vi "Image to base64_v2.vi"() -> ()   [LabVIEW 2017]
uses:
  <vilib>/wsapi/NI_WebServices.lvlib
panel:
  out "Decoded image":picture
  out "string out (base64-encoded)":string
  out "Original image":picture
  in  "path to JPEG file":path=path "E:/UPWORK/darknet/labview-meet-yolo/samples/001.jpg"
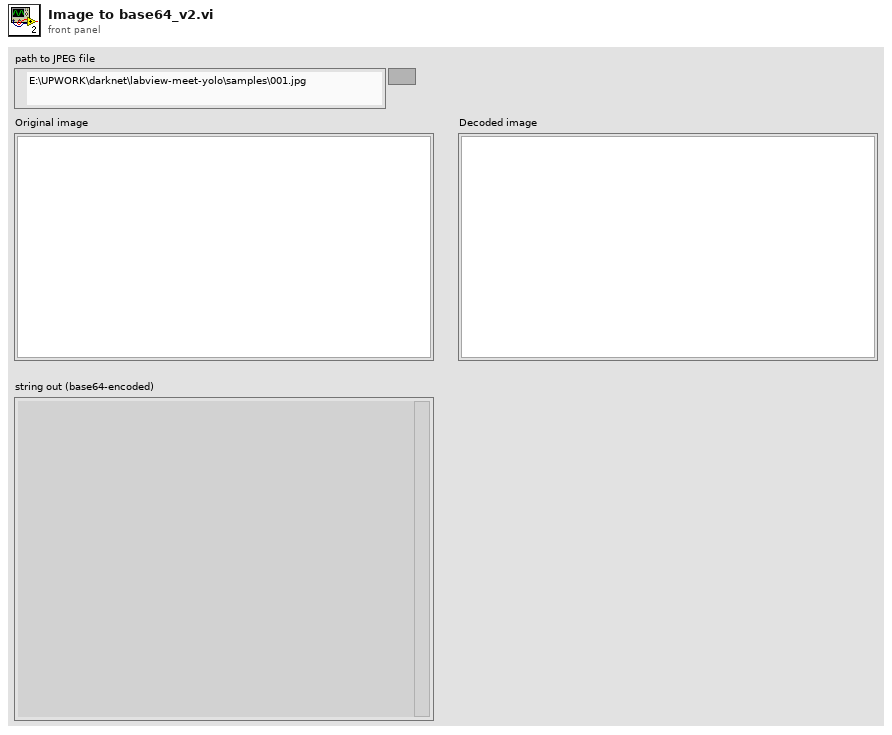
[diagram p1: front panel]
types:
  T1 = typedef "imagedata.ctl" = cluster{"image type":i32, "image depth":i32, "image":u8[], "mask":u8[], "colors":u32[], "Rectangle":cluster{"left":i16, "top":i16, "right":i16, "bottom":i16}}
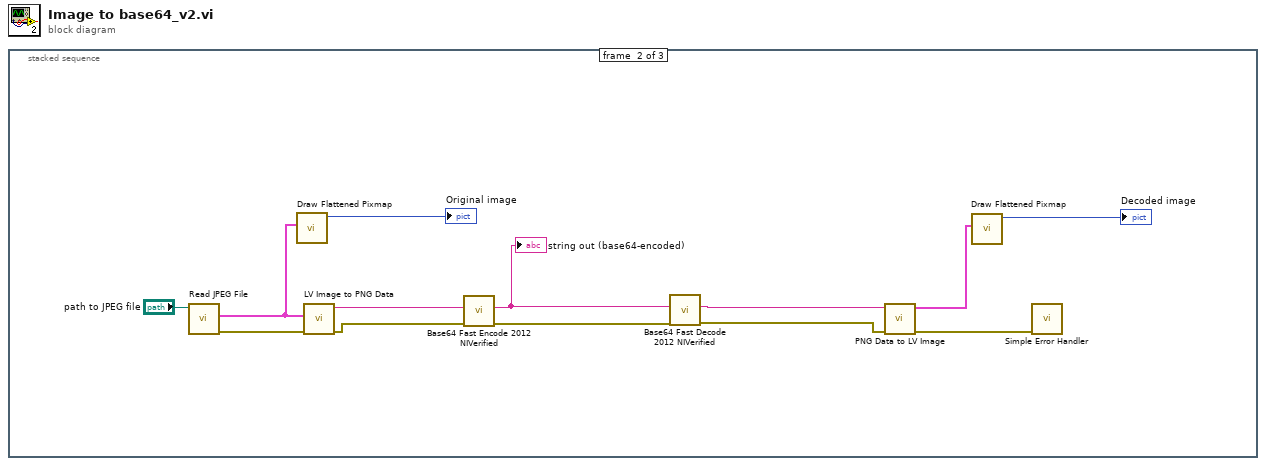
[diagram p0: block diagram]
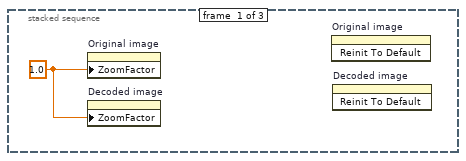
[diagram p2: hidden frame]
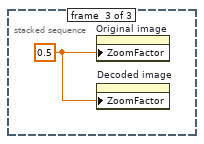
[diagram p3: hidden frame]
diagram:
  n1 = stacked-sequence {
    frame #0 {
      w1 = sgl 1.0 ("Zoom Factor")
      n2 = property on="Original image" class="Pict"("ZoomFactor"=w1) -> ()  [unwired: 2 in, 2 out]
      n3 = property on="Decoded image" class="Pict"("ZoomFactor"=w1) -> ()  [unwired: 2 in, 2 out]
      n4 = invoke on="Original image" class="Pict" method="Reinit To Default"() -> ()  [unwired: 3 in, 3 out]
      n5 = invoke on="Decoded image" class="Pict" method="Reinit To Default"() -> ()  [unwired: 3 in, 3 out]
    }
    frame #1 {
      n6 = call <vilib>:"Read JPEG File.vi"("path to JPEG file"="path to JPEG file") -> ("error out"=w13:errorcluster, "image data"=w11:T1)  [unwired: 8 in, 1 out]
      n7 = call <vilib>:"Draw Flattened Pixmap.vi"("image data"=w11) -> ("new picture"=→"Original image":picture)  [unwired: 8 in]
      n8 = call <vilib>:"LV Image to PNG Data.vi"("error in (no error)"=w13, "image data"=w11) -> ("error out"=w9:errorcluster, "png data"=w10:string)  [unwired: 8 in]
      n9 = call "Base64 Fast Encode 2012 NIVerified.vi"("error in (no error)"=w9, "string in (not encoded)"=w10) -> ("error out"=w7:errorcluster, "string out (base64-encoded)"=w8:string)  [unwired: 8 in]
      "string out (base64-encoded)" <- w8
      n10 = call "Base64 Fast Decode 2012 NIVerified.vi"("error in (no error)"=w7, "string in (base64-encoded)"=w8) -> ("error out"=w5:errorcluster, "string out (decoded)"=w6:string)  [unwired: 8 in]
      n11 = call <vilib>:"PNG Data to LV Image.vi"("error in (no error)"=w5, "png data"=w6) -> ("error out"=w3:errorcluster, "image data"=w4:T1)  [unwired: 8 in]
      n12 = call <vilib>:"Draw Flattened Pixmap.vi"("image data"=w4) -> ("new picture"=→"Decoded image":picture)  [unwired: 8 in]
      n13 = call <vilib>:"Simple Error Handler.vi"("error in (no error)"=w3) -> ()  [unwired: 4 in, 5 out]
    }
    frame #2 {
      w15 = sgl 0.5 ("Zoom Factor")
      n14 = property on="Original image" class="Pict"("ZoomFactor"=w15) -> ()  [unwired: 2 in, 2 out]
      n15 = property on="Decoded image" class="Pict"("ZoomFactor"=w15) -> ()  [unwired: 2 in, 2 out]
    }
  }
